vi "Create Sum Handles.vi"(8 "error in (no error)":errorcluster, 10 "Names":string[](array[string]), 11 "TwinCAT ADS in":refnum<class "TwinCAT ADS.lvclass">) -> (0 "error out":errorcluster, 1 "Handles":u32[](array[numeric]), 3 "TwinCAT ADS out":refnum<class "TwinCAT ADS.lvclass">)   [LabVIEW 2018, in "TwinCAT ADS.lvclass"]
uses:
  TwinCAT ADS.lvclass
  TwinCAT.Ads
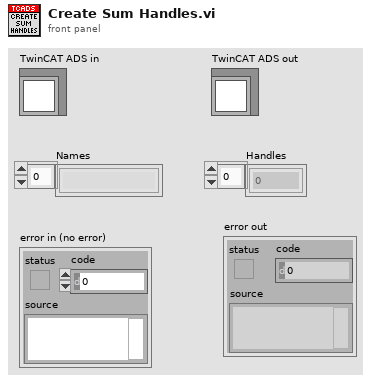
[diagram p1: front panel]
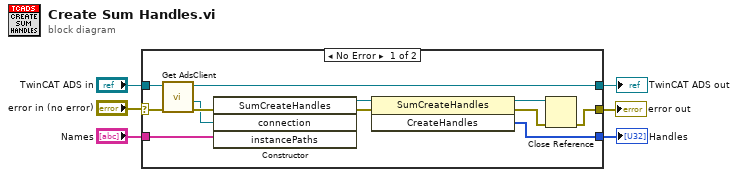
[diagram p0: block diagram]
diagram:
  n1 = case shown="No Error" "error in (no error)" {
    selector: "error in (no error)" -> [w14 w20]
    tunnel: [w7 w20] -> w5
    tunnel: [w11 w19] -> w3
    tunnel: "TwinCAT ADS in" -> [w17 w19]
    tunnel: "Names" -> [w13 _]
    tunnel: [w10 _] -> w1
    frame No Error {
      n2 = call-dynamic "Get AdsClient.vi"("error in (no error)"=w14, "TwinCAT ADS in"=w17) -> ("error out"=w16:errorcluster, ".NET TcAdsClient refnum"=w15:refnum<k24>, "TwinCAT ADS out"=w11:refnum<class "TwinCAT ADS.lvclass">)  [unwired: 7 in]
      n3 = constructor class="SumCreateHandles"(error in=w16, "connection"=w15, "instancePaths"=w13) -> (reference out=w12:refnum<k24>, error out=w18:errorcluster)  [unwired: 2 in, 3 out]
      n4 = invoke class="SumCreateHandles" method="CreateHandles"(reference=w12, error in=w18) -> (reference out=w8:refnum<k24>, error out=w9:errorcluster, "CreateHandles"=w10:u32[])  [unwired: 1 in]
      n5 = Close Reference(reference=w8, error in (no error)=w9) -> (error out=w7:errorcluster)
    }
    frame Error {
    }
  }
  "error out" <- w5
  "TwinCAT ADS out" <- w3
  "Handles" <- w1
